vi "Compare two Ranges.vi"(8 "Lower 2":dbl, 9 "Upper 2":dbl, 10 "Lower 1":dbl, 11 "Upper 1":dbl) -> (1 "Lower":dbl, 2 "Upper":dbl, 3 "In Range":bool)   [LabVIEW 2010]
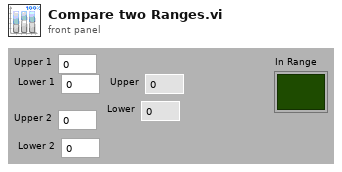
[diagram p1: front panel]
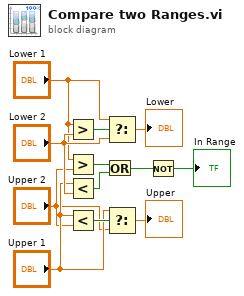
[diagram p0: block diagram]
diagram:
  n1 = Greater?(x="Lower 1", y="Lower 2") -> (0:w8:bool)
  n2 = Greater?(x="Lower 1", y="Upper 2") -> (0:w12:bool)
  n3 = Less?(x="Upper 1", y="Lower 2") -> (x < y?=w11:bool)
  n4 = Less?(x="Upper 1", y="Upper 2") -> (x < y?=w6:bool)
  n5 = Or(x=w12, y=w11) -> (x .or. y?=w10:bool)
  n6 = Select(t="Lower 1", s=w8, f="Lower 2") -> (s? t:f=→"Lower":dbl)
  n7 = Select(t="Upper 1", s=w6, f="Upper 2") -> (s? t:f=→"Upper":dbl)
  n8 = Not(x=w10) -> (.not. x?=→"In Range":bool)
